vi "Format RF Power.vi"(11 "RF Power In":string) -> (3 "Formatted RF Power":string)   [LabVIEW 2016, in "QPA TCF Parser.lvlib" / "QPA TCF Parser.lvclass"]
uses:
  QPA TCF Parser.lvclass
  <vilib>/Analysis/1siggen.llb/Ramp Pattern by Delta.vi
  <vilib>/Analysis/NI_AALBase.lvlib
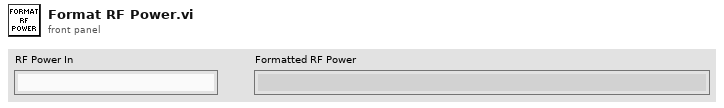
[diagram p1: front panel]
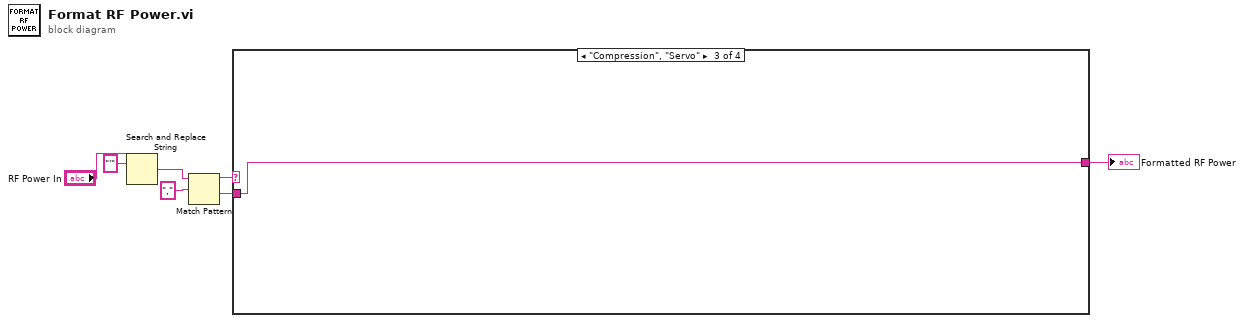
[diagram p0: block diagram]
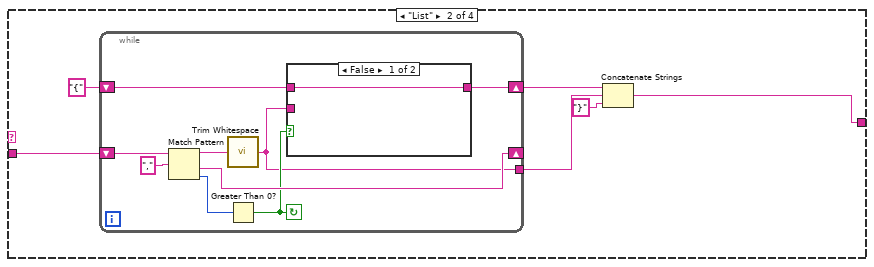
[diagram p3: hidden frame]
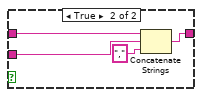
[diagram p4: hidden frame]
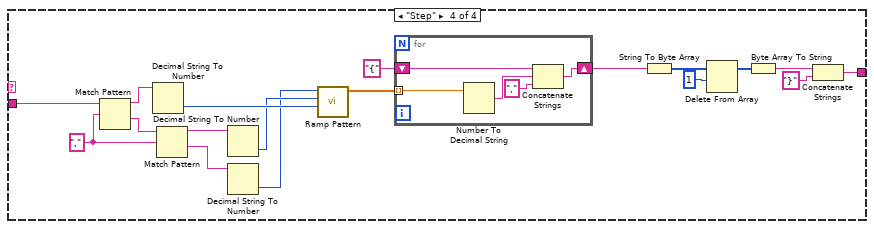
[diagram p5: hidden frame]
diagram:
  n1 = Search and Replace String(input string="RF Power In", search string="'") -> (result string=w3:string)  [unwired: 6 in, 3 out]
  n2 = Match Pattern(string=w3, regular expression=",") -> (before substring=w7:string, after substring=w5:string)  [unwired: 1 in, 2 out]
  n3 = case shown="\"Compression\", \"Servo\"" w7 {
    selector: w7 -> [w8 _ _ _]
    tunnel: [w8 w11 w29 w33] -> w4
    tunnel: w5 -> [_ w14 w29 w32]
    frame "0", Default {
    }
    frame "List" {
      n4 = while {
        shift-right: [w19] -> w12
        shift-left: "{" -> [w20]
        shift-right: [w18] -> _
        shift-left: w14 -> [w22]
        tunnel: [w15] -> w9
        stop <- w17 continue-if-true
        n5 = Match Pattern(string=w22, regular expression=",") -> (before substring=w16:string, after substring=w18:string, offset past match=w23:i32)  [unwired: 1 in, 1 out]
        n6 = call <vilib>:"Trim Whitespace.vi"("string"=w16) -> ("trimmed string"=w15:string)  [unwired: 1 in]
        n7 = Greater Than 0?(x=w23) -> (x > 0?=w17:bool)
        n8 = case shown="False" w17 {
          tunnel: w20 -> [w24 w28]
          tunnel: [w24 w27] -> w19
          tunnel: w15 -> [_ w25]
          frame False {
          }
          frame True {
            n9 = Concatenate Strings(w28, w25, "," ("string")) -> (w27:string)
          }
        }
      }
      n10 = Concatenate Strings(w12, w9, "}" ("string")) -> (w11:string)
    }
    frame "Compression", "Servo" {
    }
    frame "Step" {
      w46 = "," ("regular expression")
      n11 = Match Pattern(string=w32, regular expression=w46) -> (before substring=w45:string, after substring=w47:string)  [unwired: 1 in, 2 out]
      n12 = Decimal String To Number(string=w45) -> (number=w42:i32)  [unwired: 2 in, 1 out]
      n13 = Match Pattern(string=w47, regular expression=w46) -> (before substring=w44:string, after substring=w43:string)  [unwired: 1 in, 2 out]
      n14 = Decimal String To Number(string=w44) -> (number=w31:i32)  [unwired: 2 in, 1 out]
      n15 = Decimal String To Number(string=w43) -> (number=w30:i32)  [unwired: 2 in, 1 out]
      n16 = call-poly <vilib>:"Ramp Pattern.vi"("start"=w42, "end"=w31, "delta"=w30) -> ("Ramp Pattern"=w41:dbl[])  [unwired: 6 in, 2 out]
      n17 = for {
        tunnel: w41 -> [w52] mode=indexing
        shift-right: [w48] -> w39
        shift-left: "{" -> [w51]
        n18 = Number To Decimal String(number=w52) -> (decimal integer string=w50:string)  [unwired: 1 in]
        n19 = Concatenate Strings(w51, w50, "," ("string")) -> (w48:string)
      }
      n20 = String To Byte Array(string=w39) -> (unsigned byte array=w38:u8[])
      n21 = Delete From Array(array=w38, length=1) -> (array with subset deleted=w36:u8[])  [unwired: 1 in, 1 out]
      n22 = Byte Array To String(unsigned byte array=w36) -> (string=w34:string)
      n23 = Concatenate Strings(w34, "}" ("string")) -> (w33:string)
    }
  }
  "Formatted RF Power" <- w4
